vi "GetFrontPanel.vi"(8 "Error In":errorcluster, 11 "object in":refnum<class "Mockup_ConfigurationManager.lvclass">) -> (0 "Error Out":errorcluster, 2 "FrontPanel":refnum<class "FrontPanelControl.lvclass">, 3 "object out":refnum<class "Mockup_ConfigurationManager.lvclass">)   [LabVIEW 2021, in "Mockup_ConfigurationManager.lvclass"]
uses:
  Mockup_ConfigurationManager.lvclass
  .Externals/Library_UserInterface_FrontPanelControl/FrontPanelControl/FrontPanelControl.lvclass
panel:
  in  "Items":u16(ring)
  in  "Tree":string(tree)
  in  "Save":bool
  in  "Cancel":bool
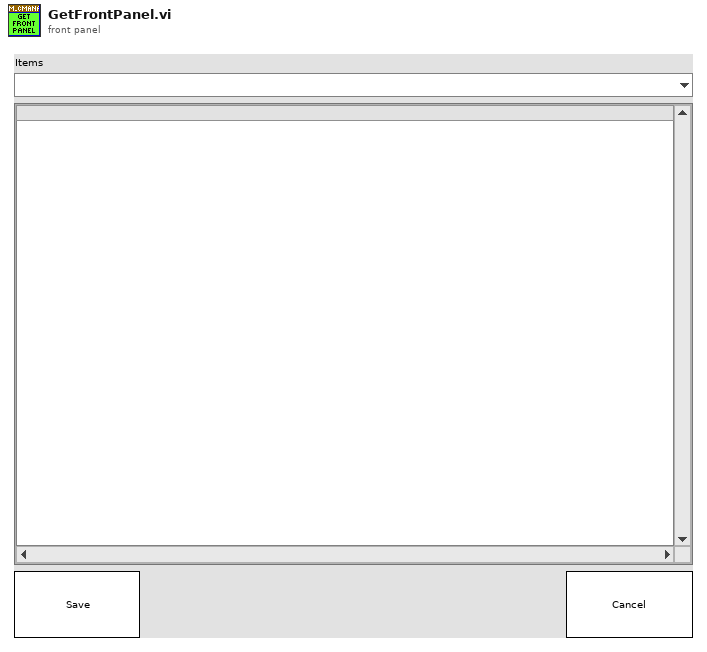
[diagram p1: front panel]
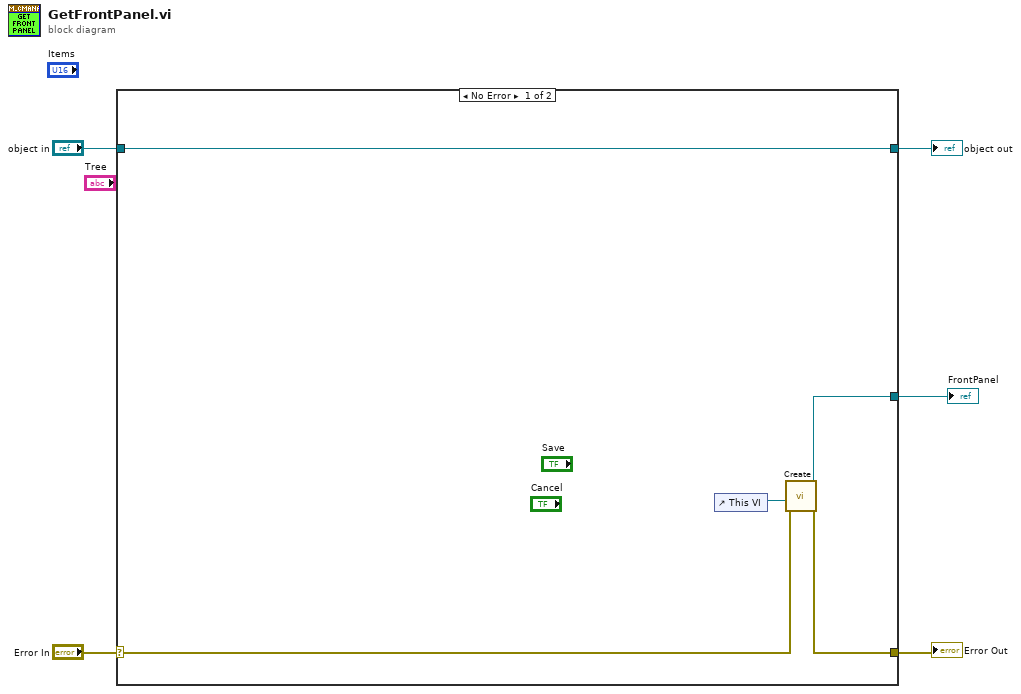
[diagram p0: block diagram]
diagram:
  n1 = case shown="No Error" "Error In" {
    selector: "Error In" -> [w8 w12]
    tunnel: [w7 w12] -> w4
    tunnel: [w10 w11] -> w2
    tunnel: "object in" -> [w10 w11]
    tunnel: [w6 _] -> w1
    frame No Error {
      n2 = control-ref of="This VI"() -> (w9:refnum<vi>)
      n3 = call "Create.vi"("Error In"=w8, "VIRef"=w9) -> ("Error Out"=w7:errorcluster, "object out"=w6:refnum<class "FrontPanelControl.lvclass">)  [unwired: 8 in]
    }
    frame Error {
    }
  }
  "Error Out" <- w4
  "object out" <- w2
  "FrontPanel" <- w1
